vi "TCP-SV Message Interpreter.vi"(8 "error in (no error)":errorcluster, 9 "Data":variant, 10 "Message":string, 11 "Guardian in":refnum<class "Guardian.lvclass">) -> (0 "error out":errorcluster, 3 "Guardian out":refnum<class "Guardian.lvclass">)   [LabVIEW 2020, in "TALOS.lvlib" / "Guardian.lvlib" / "Guardian.lvclass"]
doc: "Use this VI to send a message to the Guardian, from the outside (i.e. from a uService). For internal messages, use the Actor Framework messages system."
uses:
  Guardian.lvclass
  C:/LabVIEW Code/TALOS/talos/Ancestor/Ancestor/Ancestor.lvclass
  C:/LabVIEW Code/TALOS/builds/Actor Framework PPL/Actor Framework.lvlibp/1abvi3w/vi.lib/ActorFramework/Actor/Actor.lvclass
  Ancestor/Ancestor/Ancestor.lvclass/Ancestor.ctl
  Father of all uServices/Father of all uServices/Event Handler Items.ctl
  Classes/uService List/uService List.lvclass/uService List.ctl
  Father of all uServices/Father of all uServices Messages/Event Handler Msg/Event Handler Msg.lvclass/Event Handler Msg.ctl
  Guardian Messages/Ready to launch Msg/Ready to launch Msg.lvclass/Ready to launch Msg.ctl
  Guardian.lvclass/Guardian.ctl
  Guardian Messages/Message to uService Msg/Message to uService Msg.lvclass/Message to uService Msg.ctl
  Ancestor/Ancestor/Infinite Message Selector.ctl
  Im alive message.ctl
  Guardian Messages/Message to Other Guardian Msg/Message to Other Guardian Msg.lvclass/Message to Other Guardian Msg.ctl
  Classes/uService List/Get Queue.vi
  FGV/Error Memory/Get Error Description.vi
  Support VIs/Get PC name.vi
  Support VIs/Get Class Name.vi
  <vilib>/Utility/error.llb/Clear Errors.vi
  Support VIs/Circus Root Path.vi
  FGV/Error Memory/Error Memory Core.vi
  <vilib>/AdvancedString/Delimited String to 1D String Array.vi
  FGV/Error Memory/Error Crt Lvl checker.vi
  FGV/Error Memory/Error Memory Core.vi/40c8088d-b597-4017-91af-faa98e00292e.vi
  FGV/Error Memory/Error Memory Core.vi/d4a3ab98-063c-4e44-b43d-fbdcfe6c2be2.vi
  Support VIs/Global Memory.vi
  <vilib>/Utility/LVClass/Get LV Class Name.vi
  Support VIs/TALOS Root path.vi
  Support VIs/Read CSV worksheet.vi
  Support VIs/Global Constants.vi
  <vilib>/Utility/error.llb/General Error Handler.vi
  <vilib>/Utility/config.llb/Open Config Data.vi
  <vilib>/Utility/config.llb/Get Section Names.vi
  <vilib>/Utility/config.llb/Get Key Names.vi
  <vilib>/Utility/config.llb/Read Key.vi
  <vilib>/Utility/config.llb/Read Key (String).vi
  <vilib>/Utility/config.llb/Close Config Data.vi
  builds/Actor Framework PPL/Actor Framework.lvlibp/1abvi3w/vi.lib/ActorFramework/Message Enqueuer/Enqueue.vi
  Support VIs/Error Log.vi
  Ancestor/Ancestor/Ancestor.lvclass
  <vilib>/Comparison/Equal/Equal Functor/Equal Functor.lvclass
  builds/Actor Framework PPL/Actor Framework.lvlibp/1abvi3w/vi.lib/ActorFramework/Message Enqueuer/Message Enqueuer.lvclass
  Father of all uServices/Father of all uServices Messages/Event Handler Msg/Event Handler Msg.lvclass
  Guardian Messages/Ready to launch Msg/Ready to launch Msg.lvclass
  Guardian Messages/Message to uService Msg/Message to uService Msg.lvclass
  Guardian Messages/Message to Other Guardian Msg/Message to Other Guardian Msg.lvclass
  Classes/Guardian List/Guardian List.lvclass
  Classes/Distributed uService Map/Distributed uService Map.lvclass
  TALOS.lvlib
  Father of all uServices/Father of all uServices/Father of all uServices.lvclass
  Classes/uService List/uService List.lvclass
  builds/Actor Framework PPL/Actor Framework.lvlibp/1abvi3w/vi.lib/ActorFramework/Actor/Actor.lvclass
  Classes/Error Filter/Error Filter.lvclass
  FGV/Error Memory/Error Memory.lvlib
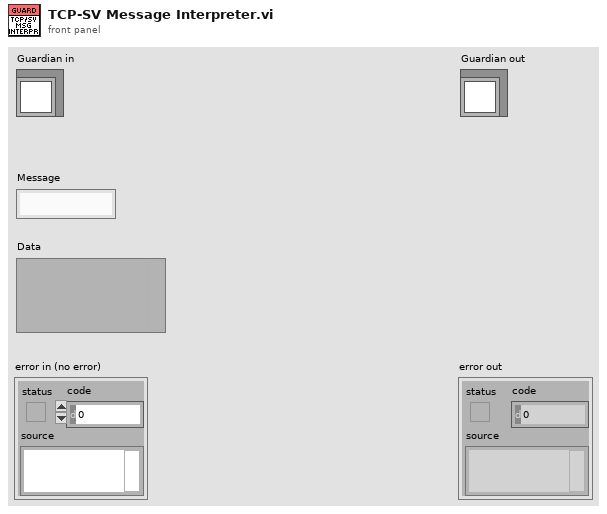
[diagram p1: front panel]
types:
  T1 = typedef "TALOS.lvlib/Father of all uServices.lvlib/Father of all uServices.lvclass/Event Handler Items.ctl" = enum16{"Button Pressed", "Shared Variable Updated", "Message", "Ready to launch?", "Safe Mode", "Start RUN", "Stop RUN"}
  T2 = typedef "TALOS.lvlib/Ancestor.lvlib/Ancestor.lvclass/Infinite Message Selector.ctl" = enum16{"Start", "Stop", "Check", "Flush (Stop all)", "Init"}
  T3 = typedef "TALOS.lvlib/Guardian.lvlib/Guardian.lvclass/Im alive message.ctl" = cluster{"ID":string, "Time":timestamp}
  T4 = cluster{"Accessors:ID":string, "All IDs":string[]}
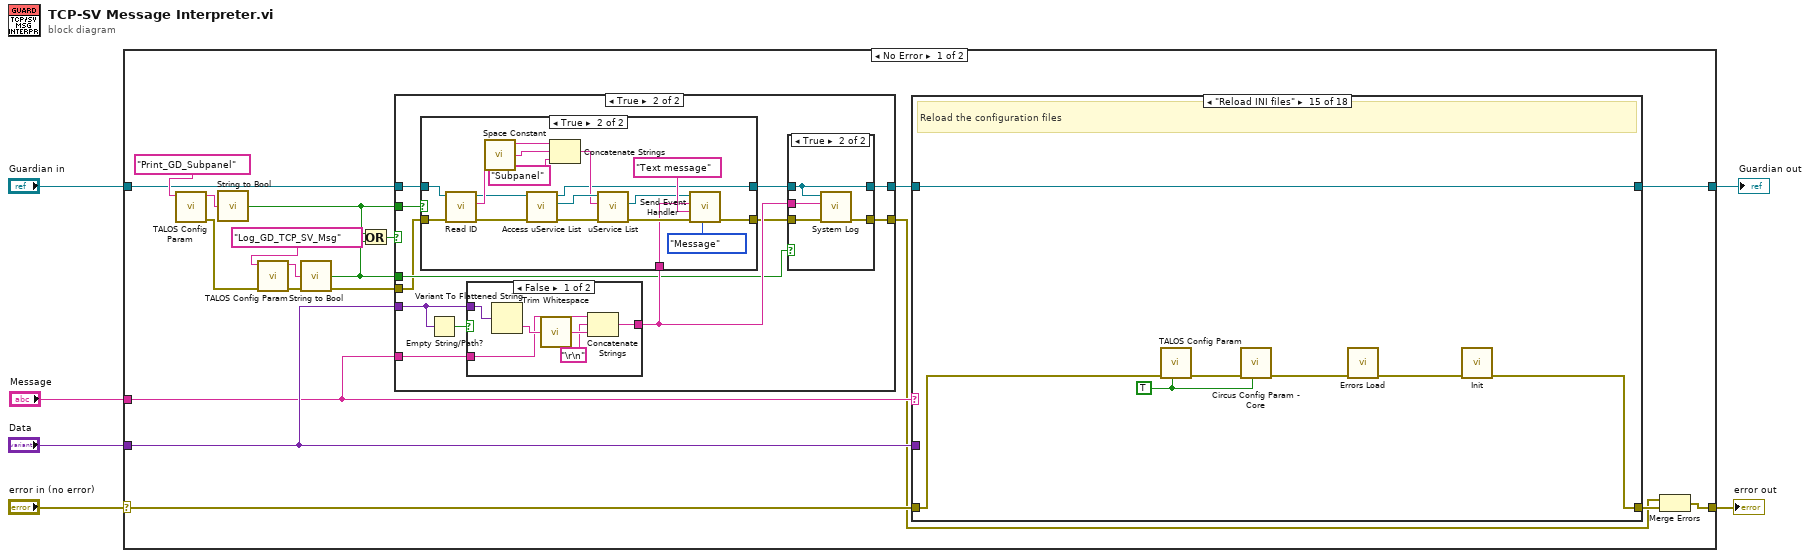
[diagram p0: block diagram]
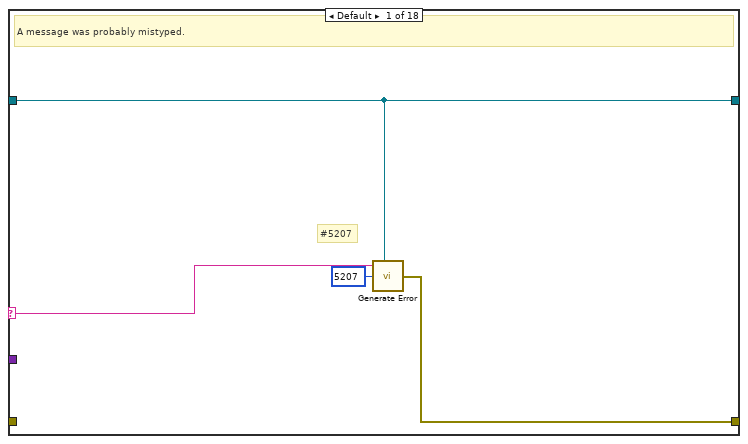
[diagram p6: hidden frame]
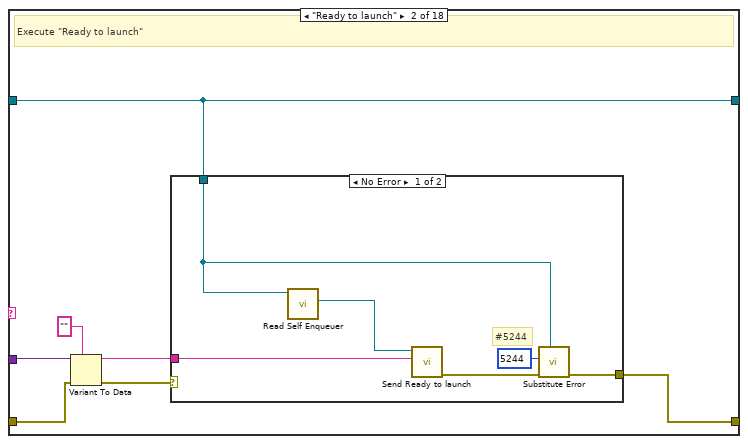
[diagram p7: hidden frame]
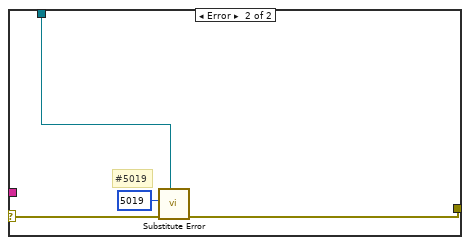
[diagram p8: hidden frame]
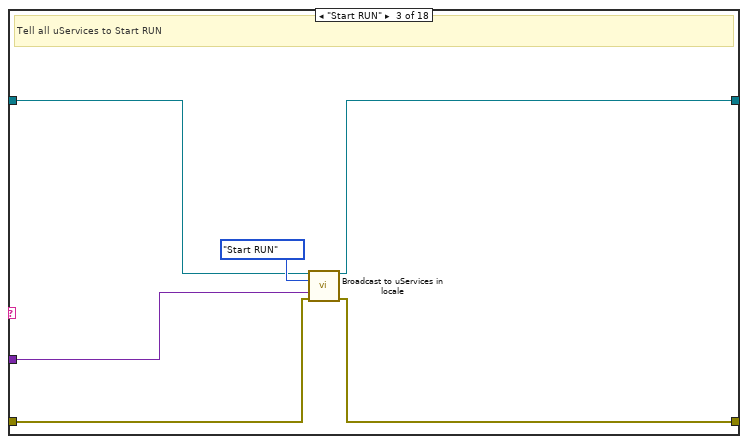
[diagram p9: hidden frame]
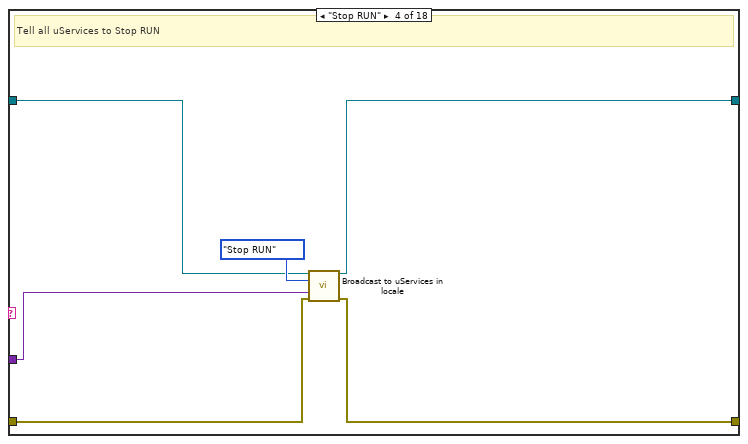
[diagram p10: hidden frame]
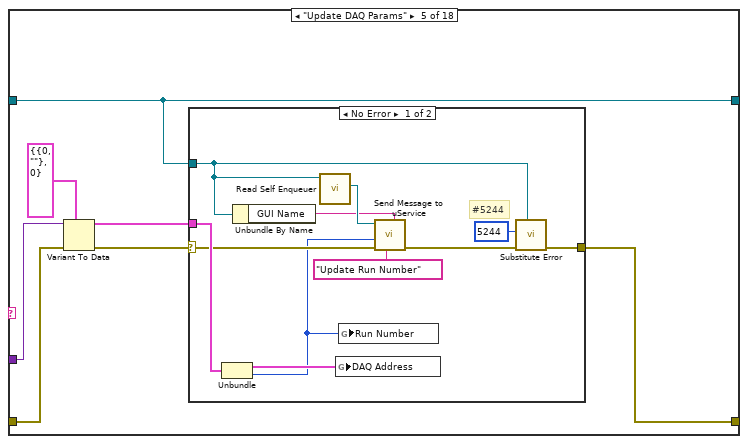
[diagram p11: hidden frame]
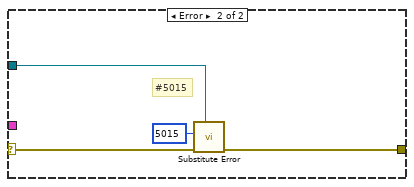
[diagram p12: hidden frame]
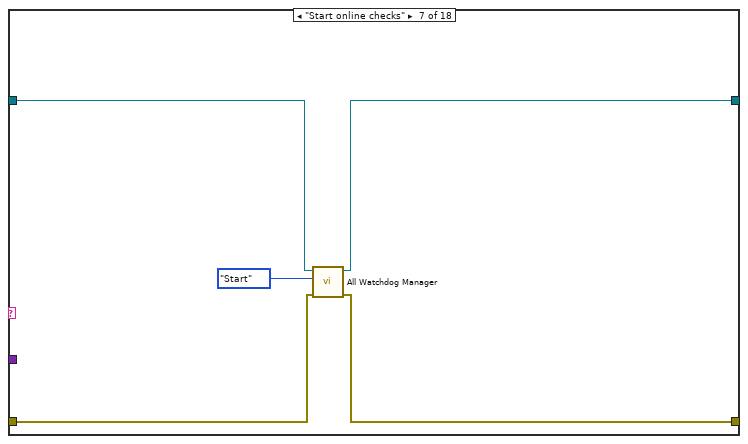
[diagram p14: hidden frame]
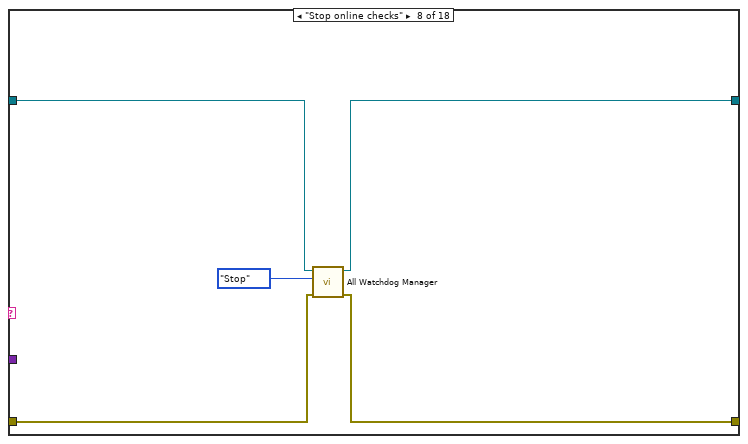
[diagram p15: hidden frame]
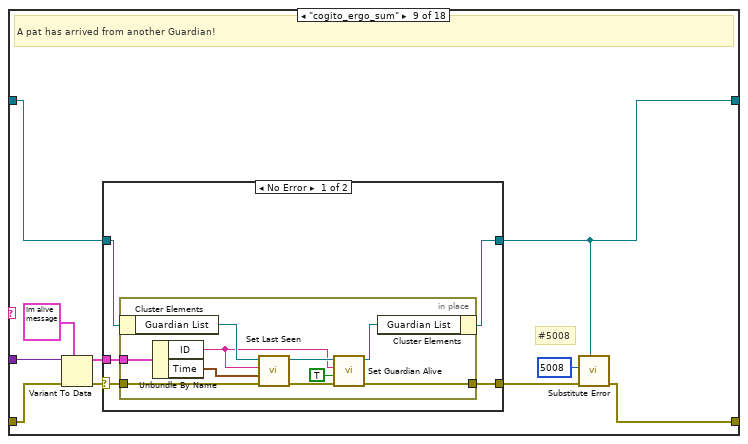
[diagram p16: hidden frame]
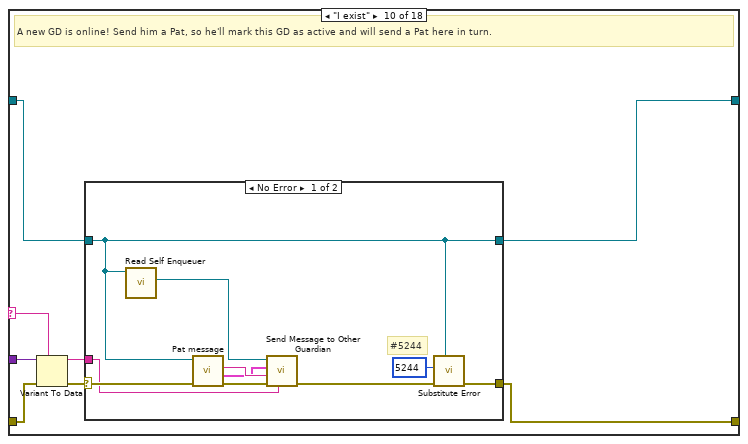
[diagram p18: hidden frame]
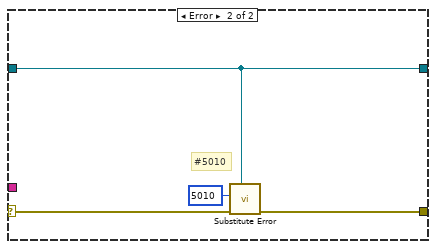
[diagram p19: hidden frame]
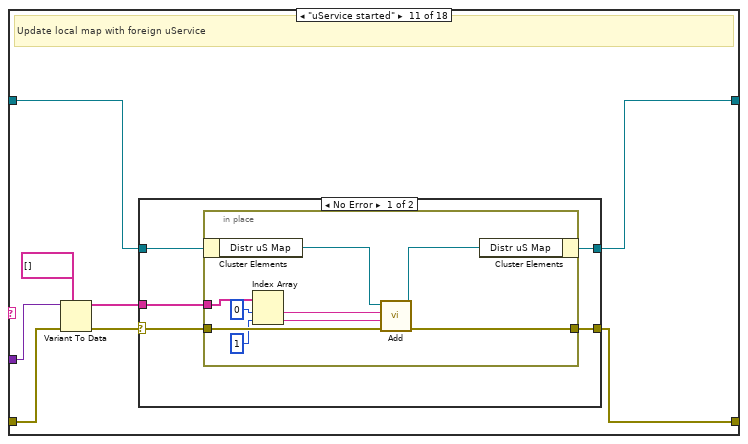
[diagram p20: hidden frame]
diagram:
  n1 = case shown="No Error" "error in (no error)" {
    selector: "error in (no error)" -> [w22 w358]
    tunnel: [w19 w358] -> w6
    tunnel: "Guardian in" -> [w15 w357]
    tunnel: [w23 w357] -> w3
    tunnel: "Data" -> [w21 _]
    tunnel: "Message" -> [w20 _]
    frame No Error {
      n2 = call "TALOS Config Param.vi"("Parameter Name"="Print_GD_Subpanel") -> ("error out"=w11:errorcluster, "Output"=w16:string)  [unwired: 9 in]
      n3 = call "String to Bool.vi"("String"=w16) -> ("Boolean"=w7:bool)
      n4 = call "TALOS Config Param.vi"("error in (no error)"=w11, "Parameter Name"="Log_GD_TCP_SV_Msg") -> ("error out"=w10:errorcluster, "Output"=w13:string)  [unwired: 8 in]
      n5 = call "String to Bool.vi"("String"=w13) -> ("Boolean"=w8:bool)
      n6 = Or(x=w7, y=w8) -> (x .or. y?=w9:bool)
      n7 = case shown="True" w9 {
        tunnel: w21 -> [_ w37]
        tunnel: w20 -> [_ w36]
        tunnel: [w25 w35] -> w18
        tunnel: w15 -> [w26 w31]
        tunnel: w7 -> [_ w30]
        tunnel: w8 -> [_ w29]
        tunnel: [w26 w28] -> w12
        tunnel: w10 -> [w25 w27]
        frame False {
        }
        frame True {
          n8 = Empty String/Path?(string/path=w37) -> (empty?=w38:bool)
          n9 = case shown="False" w38 {
            tunnel: w37 -> [w69 _]
            tunnel: w36 -> [w66 w70]
            tunnel: [w64 w70] -> w34
            frame False {
              n10 = Variant To Flattened String(Variant=w69) -> (data string=w68:string)  [unwired: 1 out]
              n11 = call <vilib>:"Trim Whitespace.vi"("string"=w68) -> ("trimmed string"=w67:string)  [unwired: 1 in]
              n12 = Concatenate Strings(w66, "\r\n", w67) -> (w64:string)
            }
            frame True {
            }
          }
          n13 = case shown="True" w30 {
            tunnel: w34 -> [_ w54]
            tunnel: [w40 w47] -> w33
            tunnel: [w39 w46] -> w32
            tunnel: w31 -> [w40 w43]
            tunnel: w27 -> [w39 w42]
            frame False {
            }
            frame True {
              n14 = call "Read ID.vi"("error in (no error)"=w42, "Ancestor in"=w43) -> ("error out"=w41:errorcluster, "ID"=w45:string, "Ancestor out"=w44:refnum<class "Guardian.lvclass">)  [unwired: 7 in]
              n15 = call <vilib>:"Space Constant.vi"() -> ("String"=w48:string)
              n16 = call-dynamic "Access uService List.vi"("error in (no error)"=w41, "Ancestor in"=w44) -> ("error out"=w52:errorcluster, "uService List out"=w51:refnum<class "uService List.lvclass">, "Ancestor out"=w47:refnum<class "Guardian.lvclass">)  [unwired: 7 in]
              n17 = Concatenate Strings(w45, w48, "Subpanel" ("string")) -> (w50:string)
              n18 = call-poly "uService List.vi"("error in (no error)"=w52, "ID"=w50, "uService List in"=w51) -> ("error out"=w57:errorcluster, "uService Queue"=w53:refnum<class "Message Enqueuer.lvclass">)  [unwired: 6 in, 1 out]
              n19 = call "Send Event Handler.vi"("Event type"=Event_Handler_Items."Message", "error in (no error)"=w57, "Item Name"="Text message" ("Message"), "Data"=w54, "Message Enqueuer"=w53) -> ("error out"=w46:errorcluster)  [unwired: 5 in, 1 out]
            }
          }
          n20 = case shown="True" w29 {
            tunnel: [w59 w63] -> w35
            tunnel: w34 -> [_ w62]
            tunnel: w33 -> [w58 w60]
            tunnel: w32 -> [w59 w61]
            tunnel: [w58 w60] -> w28
            frame False {
            }
            frame True {
              n21 = call "System Log.vi"("error in (no error)"=w61, "Text to log"=w62, "Object in"=w60) -> ("error out"=w63:errorcluster)  [unwired: 8 in]
            }
          }
        }
      }
      n22 = case shown="\"Reload INI files\"" w20 {
        selector: w20 -> [w72 _ _ _ _ _ _ _ _ w166 _ _ _ _ _ w316 _ _]
        tunnel: [w73 w80 w95 w101 w105 w126 w129 w134 w139 w165 w187 w213 w239 w268 w302 w310 w324 w349] -> w24
        tunnel: w21 -> [_ w79 w92 w98 w110 _ _ _ w147 w172 w192 w218 w244 w272 _ w314 _ w356]
        tunnel: w12 -> [w71 w81 w93 w99 w106 w127 w132 w137 w142 w168 w194 w220 w246 w274 w308 w309 w323 w347]
        tunnel: [w71 w81 w96 w102 w106 w127 w131 w136 w140 w167 w193 w219 w245 w273 w308 w309 w321 w348] -> w23
        tunnel: w22 -> [_ w78 w94 w100 w104 w126 w128 w133 w145 w171 w191 w217 w243 w271 w307 w313 w325 w350]
        frame Default {
          # "#5207"
          # "A message was probably mistyped."
          n23 = call "Generate Error.vi"("Optional String"=w72, "Class"=w71, "Error Code"=5207) -> ("error out"=w73:errorcluster)  [unwired: 4 in]
        }
        frame "Ready to launch" {
          # "Execute \"Ready to launch\""
          n24 = Variant To Data(error in=w78, type="", Variant=w79) -> (data=w75:string, error out=w76:errorcluster)
          n25 = case shown="No Error" w76 {
            selector: w76 -> [_ w90]
            tunnel: w81 -> [w82 w91]
            tunnel: [w83 w89] -> w80
            tunnel: w75 -> [w86 _]
            frame No Error {
              # "#5244"
              n26 = call "Read Self Enqueuer.vi"("Actor"=w82) -> ("Self Enqueuer"=w87:refnum<class "Message Enqueuer.lvclass">)  [unwired: 10 in]
              n27 = call "Send Ready to launch.vi"("GUID"=w86, "Message Enqueuer"=w87) -> ("error out"=w84:errorcluster)  [unwired: 8 in, 1 out]
              n28 = call "Substitute Error.vi"("LabVIEW Object"=w82, "error in (no error)"=w84, "Error Code"=5244) -> ("error out"=w83:errorcluster)  [unwired: 8 in]
            }
            frame Error {
              # "#5019"
              n29 = call "Substitute Error.vi"("LabVIEW Object"=w91, "error in (no error)"=w90, "Error Code"=5019) -> ("error out"=w89:errorcluster)  [unwired: 8 in]
            }
          }
        }
        frame "Start RUN" {
          # "Tell all uServices to Start RUN"
          n30 = call "Broadcast to uServices in locale.vi"("Guardian in"=w93, "Event type"=Event_Handler_Items."Start RUN", "Data"=w92, "error in (no error)"=w94) -> ("Guardian out"=w96:refnum<class "Guardian.lvclass">, "error out"=w95:errorcluster)  [unwired: 10 in]
        }
        frame "Stop RUN" {
          # "Tell all uServices to Stop RUN"
          n31 = call "Broadcast to uServices in locale.vi"("Guardian in"=w99, "Event type"=Event_Handler_Items."Stop RUN", "Data"=w98, "error in (no error)"=w100) -> ("Guardian out"=w102:refnum<class "Guardian.lvclass">, "error out"=w101:errorcluster)  [unwired: 10 in]
        }
        frame "Update DAQ Params" {
          n32 = Variant To Data(error in=w104, type=cluster{cluster{u16, string}, i32} {{0, ""}, 0}, Variant=w110) -> (data=w108:cluster{cluster{u16, string}, i32}, error out=w107:errorcluster)
          n33 = case shown="No Error" w107 {
            selector: w107 -> [w118 w125]
            tunnel: w108 -> [w119 _]
            tunnel: w106 -> [w112 w123]
            tunnel: [w111 w124] -> w105
            frame No Error {
              # "#5244"
              n34 = Unbundle(w119) -> (w116:cluster{u16, string}, w115:i32)
              n35 = Unbundle By Name(w112) -> ("GUI Name"=w120:string)
              n36 = call "Read Self Enqueuer.vi"("Actor"=w112) -> ("Self Enqueuer"=w121:refnum<class "Message Enqueuer.lvclass">)  [unwired: 10 in]
              n37 = global write "Global Memory.vi" "DAQ Address"(w116) -> ()
              n38 = global write "Global Memory.vi" "Run Number"(w115) -> ()
              n39 = call "Send Message to uService.vi"("uService ID"=w120, "Message"="Update Run Number", "error in (no error)"=w118, "Data"=w115, "Message Enqueuer"=w121) -> ("error out"=w113:errorcluster)  [unwired: 5 in, 1 out]
              n40 = call "Substitute Error.vi"("LabVIEW Object"=w112, "error in (no error)"=w113, "Error Code"=5244) -> ("error out"=w111:errorcluster)  [unwired: 8 in]
            }
            frame Error {
              # "#5015"
              n41 = call "Substitute Error.vi"("LabVIEW Object"=w123, "error in (no error)"=w125, "Error Code"=5015) -> ("error out"=w124:errorcluster)  [unwired: 8 in]
            }
          }
        }
        frame "Text Message" {
          # "For testing purpouses"
        }
        frame "Start online checks" {
          n42 = call "All Watchdog Manager.vi"("error in (no error)"=w128, "Infinite Message Selector"=Infinite_Message_Selector."Start", "Guardian in"=w132) -> ("error out"=w129:errorcluster, "Guardian out"=w131:refnum<class "Guardian.lvclass">)  [unwired: 6 in, 1 out]
        }
        frame "Stop online checks" {
          n43 = call "All Watchdog Manager.vi"("error in (no error)"=w133, "Infinite Message Selector"=Infinite_Message_Selector."Stop", "Guardian in"=w137) -> ("error out"=w134:errorcluster, "Guardian out"=w136:refnum<class "Guardian.lvclass">)  [unwired: 6 in, 1 out]
        }
        frame "cogito_ergo_sum" {
          # "#5008"
          # "A pat has arrived from another Guardian!"
          n44 = Variant To Data(error in=w145, type=T3 {"ID"="", "Time"=timestamp(0 s since 1904-01-01)} ("cluster"), Variant=w147) -> (data=w144:T3, error out=w143:errorcluster)
          n45 = case shown="No Error" w143 {
            selector: w143 -> [w149 w163]
            tunnel: w144 -> [w150 _]
            tunnel: w142 -> [w152 w164]
            tunnel: [w151 w164] -> w140
            tunnel: [w148 w163] -> w141
            frame No Error {
              n46 = in-place {
                in-place-border: w150 -> [w161]
                in-place-border: w149 -> [w159]
                in-place-border: [w155] -> w148
                n47 = in-place-cluster #1(w152) -> ("Guardian List"=w162:refnum<class "Guardian List.lvclass">)
                n48 = Unbundle By Name(w161) -> ("ID"=w154:string, "Time"=w160:timestamp)
                n49 = call-dynamic "Set Last Seen.vi"("error in (no error)"=w159, "Last Seen"=w160, "ID"=w154, "Guardian List in"=w162) -> ("error out"=w156:errorcluster, "Guardian List out"=w158:refnum<class "Guardian List.lvclass">)  [unwired: 6 in]
                n50 = call-dynamic "Set Guardian Alive.vi"("error in (no error)"=w156, "Alive"=TRUE, "ID"=w154, "Guardian List in"=w158) -> ("error out"=w155:errorcluster, "Guardian List out"=w157:refnum<class "Guardian List.lvclass">)  [unwired: 6 in]
                n51 = in-place-cluster #1("Guardian List"=w157) -> (w151:refnum<class "Guardian.lvclass">)
              }
            }
            frame Error {
            }
          }
          n52 = call "Substitute Error.vi"("LabVIEW Object"=w140, "error in (no error)"=w141, "Error Code"=5008) -> ("error out"=w139:errorcluster)  [unwired: 8 in]
        }
        frame "I exist" {
          # "A new GD is online! Send him a Pat, so he'll mark this GD as active and will send a Pat here in turn."
          n53 = Variant To Data(error in=w171, type=w166, Variant=w172) -> (data=w170:string, error out=w169:errorcluster)
          n54 = case shown="No Error" w169 {
            selector: w169 -> [w181 w185]
            tunnel: w170 -> [w180 _]
            tunnel: w168 -> [w174 w186]
            tunnel: [w174 w186] -> w167
            tunnel: [w173 w183] -> w165
            frame No Error {
              # "#5244"
              n55 = call "Read Self Enqueuer.vi"("Actor"=w174) -> ("Self Enqueuer"=w182:refnum<class "Message Enqueuer.lvclass">)  [unwired: 10 in]
              n56 = call "Pat message.vi"("error in (no error)"=w181, "Guardian in"=w174) -> ("error out"=w177:errorcluster, "Data"=w178:T3, "Message name"=w179:string)  [unwired: 6 in, 1 out]
              n57 = call "Send Message to Other Guardian.vi"("Guardian ID"=w180, "error in (no error)"=w177, "Message"=w179, "Data"=w178, "Message Enqueuer"=w182) -> ("error out"=w175:errorcluster)  [unwired: 5 in, 1 out]
              n58 = call "Substitute Error.vi"("LabVIEW Object"=w174, "error in (no error)"=w175, "Error Code"=5244) -> ("error out"=w173:errorcluster)  [unwired: 8 in]
            }
            frame Error {
              # "#5010"
              n59 = call "Substitute Error.vi"("LabVIEW Object"=w186, "error in (no error)"=w185, "Error Code"=5010) -> ("error out"=w183:errorcluster)  [unwired: 8 in]
            }
          }
        }
        frame "uService started" {
          # "Update local map with foreign uService"
          n60 = Variant To Data(error in=w191, type=string[] [], Variant=w192) -> (data=w188:string[], error out=w189:errorcluster)
          n61 = case shown="No Error" w189 {
            selector: w189 -> [w197 w212]
            tunnel: w194 -> [w199 w210]
            tunnel: [w198 w210] -> w193
            tunnel: w188 -> [w195 _]
            tunnel: [w196 w209] -> w187
            frame No Error {
              n62 = in-place {
                in-place-border: w197 -> [w206]
                in-place-border: [w205] -> w196
                in-place-border: w195 -> [w204]
                n63 = in-place-cluster #2(w199) -> ("Distr uS Map"=w208:refnum<class "Distributed uService Map.lvclass">)
                n64 = Index Array(array=w204, index #1=0 ("index"), index #2=1 ("index")) -> (element #1=w201:string, element #2=w200:string)
                n65 = call-dynamic "Add.vi"("error in (no error)"=w206, "uService"=w200, "Guardian"=w201, "Distributed uService Map in"=w208) -> ("error out"=w205:errorcluster, "Distributed uService Map out"=w207:refnum<class "Distributed uService Map.lvclass">)  [unwired: 5 in, 1 out]
                n66 = in-place-cluster #2("Distr uS Map"=w207) -> (w198:refnum<class "Guardian.lvclass">)
              }
            }
            frame Error {
              # "#5102"
              n67 = call "Substitute Error.vi"("LabVIEW Object"=w210, "error in (no error)"=w212, "Error Code"=5102) -> ("error out"=w209:errorcluster)  [unwired: 8 in]
            }
          }
        }
        frame "uService stopped" {
          # "Update local map with foreign uService"
          n68 = Variant To Data(error in=w217, type=string[] [], Variant=w218) -> (data=w214:string[], error out=w215:errorcluster)
          n69 = case shown="No Error" w215 {
            selector: w215 -> [w223 w238]
            tunnel: w220 -> [w225 w236]
            tunnel: [w224 w236] -> w219
            tunnel: w214 -> [w221 _]
            tunnel: [w222 w235] -> w213
            frame No Error {
              n70 = in-place {
                in-place-border: w223 -> [w232]
                in-place-border: [w231] -> w222
                in-place-border: w221 -> [w230]
                n71 = in-place-cluster #3(w225) -> ("Distr uS Map"=w234:refnum<class "Distributed uService Map.lvclass">)
                n72 = Index Array(array=w230, index #1=0 ("index"), index #2=1 ("index")) -> (element #1=w227:string, element #2=w226:string)
                n73 = call-dynamic "Remove.vi"("error in (no error)"=w232, "uService ID"=w226, "Guardian"=w227, "Distributed uService Map in"=w234) -> ("error out"=w231:errorcluster, "Distributed uService Map out"=w233:refnum<class "Distributed uService Map.lvclass">)  [unwired: 5 in, 1 out]
                n74 = in-place-cluster #3("Distr uS Map"=w233) -> (w224:refnum<class "Guardian.lvclass">)
              }
            }
            frame Error {
              # "#5102"
              n75 = call "Substitute Error.vi"("LabVIEW Object"=w236, "error in (no error)"=w238, "Error Code"=5102) -> ("error out"=w235:errorcluster)  [unwired: 8 in]
            }
          }
        }
        frame "Get uService List" {
          # "Give to the requesting Guardian the current uService List (for initialise the distributed one)"
          n76 = Variant To Data(error in=w243, type="", Variant=w244) -> (data=w240:string, error out=w241:errorcluster)
          n77 = case shown="No Error" w241 {
            selector: w241 -> [w257 w266]
            tunnel: w246 -> [w258 w264]
            tunnel: [w247 w264] -> w245
            tunnel: w240 -> [w262 _]
            tunnel: [w248 w263] -> w239
            frame No Error {
              # "#5244"
              # "requesting GD"
              n78 = call-dynamic "Access uService List.vi"("error in (no error)"=w257, "Ancestor in"=w258) -> ("error out"=w255:errorcluster, "uService List out"=w256:refnum<class "uService List.lvclass">, "Ancestor out"=w259:refnum<class "Guardian.lvclass">)  [unwired: 7 in]
              n79 = call "Get all IDs.vi"("error in (no error)"=w255, "uService List"=w256) -> ("error out"=w254:errorcluster, "All IDs"=w252:string[])  [unwired: 7 in, 1 out]
              n80 = property class="Guardian.lvclass"(reference=w259) -> (reference out=w247:refnum<class "Guardian.lvclass">, "Accessors:ID"=w253:string)  [unwired: 1 in, 1 out]
              n81 = Bundle("Accessors:ID"=w253, "All IDs"=w252) -> (w251:T4)  [unwired: 1 in]
              n82 = call "Read Self Enqueuer.vi"("Actor"=w247) -> ("Self Enqueuer"=w261:refnum<class "Message Enqueuer.lvclass">)  [unwired: 10 in]
              n83 = call "Send Message to Other Guardian.vi"("Guardian ID"=w262, "error in (no error)"=w254, "Message"="Current uService List", "Data"=w251, "Message Enqueuer"=w261) -> ("error out"=w249:errorcluster)  [unwired: 5 in, 1 out]
              n84 = call "Substitute Error.vi"("LabVIEW Object"=w247, "error in (no error)"=w249, "Error Code"=5244) -> ("error out"=w248:errorcluster)  [unwired: 8 in]
            }
            frame Error {
              # "#5102"
              n85 = call "Substitute Error.vi"("LabVIEW Object"=w264, "error in (no error)"=w266, "Error Code"=5102) -> ("error out"=w263:errorcluster)  [unwired: 8 in]
            }
          }
        }
        frame "Current uService List" {
          # "Update Distributed uService List with the list received"
          n86 = Variant To Data(error in=w271, type=cluster{"String":string, string[]} {"String"="", []}, Variant=w272) -> (data=w269:cluster{"String":string, string[]}, error out=w270:errorcluster)
          n87 = case shown="No Error" w270 {
            selector: w270 -> [w277 w301]
            tunnel: w274 -> [w279 w299]
            tunnel: [w275 w299] -> w273
            tunnel: w269 -> [w278 _]
            tunnel: [w276 w298] -> w268
            frame No Error {
              n88 = in-place {
                in-place-border: w278 -> [w289]
                in-place-border: w277 -> [w287]
                in-place-border: [w282] -> w276
                n89 = in-place-cluster #4(w279) -> ("Distr uS Map"=w291:refnum<class "Distributed uService Map.lvclass">, "Guardian List"=w284:refnum<class "Guardian List.lvclass">)
                n90 = Unbundle(w289) -> ("String"=w285:string, w288:string[])
                n91 = for {
                  shift-right: [w296] -> w290
                  shift-left: w291 -> [w297]
                  tunnel: w285 -> [w295]
                  tunnel: w288 -> [w294] mode=indexing
                  shift-right: [w292] -> w286
                  shift-left: w287 -> [w293]
                  n92 = call-dynamic "Add.vi"("error in (no error)"=w293, "uService"=w294, "Guardian"=w295, "Distributed uService Map in"=w297) -> ("error out"=w292:errorcluster, "Distributed uService Map out"=w296:refnum<class "Distributed uService Map.lvclass">)  [unwired: 5 in, 1 out]
                }
                n93 = call-dynamic "Set uS List Received.vi"("uS List Received"=TRUE, "ID"=w285, "Guardian List in"=w284) -> ("error out"=w281:errorcluster, "Guardian List out"=w283:refnum<class "Guardian List.lvclass">)  [unwired: 7 in]
                n94 = in-place-cluster #4("Distr uS Map"=w290, "Guardian List"=w283) -> (w275:refnum<class "Guardian.lvclass">)
                n95 = Merge Errors(w286, w281) -> (w282:errorcluster)
              }
            }
            frame Error {
              # "#5102"
              n96 = call "Substitute Error.vi"("LabVIEW Object"=w299, "error in (no error)"=w301, "Error Code"=5102) -> ("error out"=w298:errorcluster)  [unwired: 8 in]
            }
          }
        }
        frame "Reload INI files" {
          w305 = TRUE ("Load")
          # "Reload the configuration files"
          n97 = call "TALOS Config Param.vi"("Load"=w305, "error in (no error)"=w307) -> ("error out"=w306:errorcluster)  [unwired: 8 in, 1 out]
          n98 = call "Circus Config Param - Core.vi"("Load"=w305, "error in (no error)"=w306) -> ("error out"=w304:errorcluster)  [unwired: 8 in, 1 out]
          n99 = call "Errors Load.vi"("error in (no error)"=w304) -> ("error out"=w303:errorcluster)  [unwired: 10 in]
          n100 = call "Init.vi"("error in (no error)"=w303) -> ("error out"=w302:errorcluster)  [unwired: 10 in]
        }
        frame "Change Run LED color", "Reset Run LED", "Run Stopped with Errors", "Update Error Listbox", "Update Kasli Log", "Update Run Status" {
          # "#5244"
          n101 = Unbundle By Name(w309) -> ("GUI Name"=w317:string)
          n102 = call "Read Self Enqueuer.vi"("Actor"=w309) -> ("Self Enqueuer"=w318:refnum<class "Message Enqueuer.lvclass">)  [unwired: 10 in]
          n103 = call "Send Message to uService.vi"("uService ID"=w317, "Message"=w316, "error in (no error)"=w313, "Data"=w314, "Locale?"=TRUE, "Message Enqueuer"=w318) -> ("error out"=w311:errorcluster)  [unwired: 4 in, 1 out]
          n104 = call "Substitute Error.vi"("LabVIEW Object"=w309, "error in (no error)"=w311, "Error Code"=5244) -> ("error out"=w310:errorcluster)  [unwired: 8 in]
        }
        frame "Update from GIT" {
          n105 = flat-sequence {
            tunnel: w325 -> [_]
            tunnel: [w326] -> w319
            tunnel: w323 -> [w331]
            tunnel: [w330] -> w320
            tunnel: w323 -> [w345]
            tunnel: [w344] -> w322
            tunnel: [w343] -> w321
            frame #0 {
              n106 = for {
                tunnel: i32[] [5004, 5005] ("Error Code") -> [w329] mode=indexing
                tunnel: [w328] -> w326 mode=indexing
                n107 = call "Add.vi"("Error Code"=w329) -> ("error out"=w328:errorcluster)  [unwired: 10 in]
              }
            }
            frame #1 {
              n108 = global read "Global Constants.vi" "Local"() -> (w335:bool)
              n109 = call "Is in Packed Library.vi"() -> ("error out"=w336:errorcluster, "Is In Packed Library"=w333:bool)  [unwired: 10 in]
              n110 = Not(x=w333) -> (.not. x?=w334:bool)
              n111 = Or(x=w335, y=w334) -> (x .or. y?=w332:bool)
              n112 = case shown="False" w332 {
                tunnel: w336 -> [w339 w342]
                tunnel: [w338 w341] -> w330
                tunnel: w331 -> [w337 _]
                frame False {
                  n113 = call "Launch Update from Git.vi"("error in (no error)"=w339, "Guardian in"=w337) -> ("error out"=w338:errorcluster)  [unwired: 8 in, 1 out]
                }
                frame True {
                  n114 = call "Temporised Pop-up Window.vi"("error in (no error)"=w342, "Text"="I'm dying!") -> ("error out"=w341:errorcluster)  [unwired: 9 in]
                }
              }
            }
            frame #2 {
              n115 = call "System shutdown.vi"("Guardian in"=w345) -> ("error out"=w344:errorcluster, "Guardian out"=w343:refnum<class "Guardian.lvclass">)  [unwired: 9 in]
            }
          }
          n116 = Merge Errors(w322, w320, w319) -> (w324:errorcluster)
        }
        frame "uServices Safe Mode" {
          w354 = TRUE
          n117 = Variant To Data(type=w354, Variant=w356) -> (data=w353:bool, error out=w355:errorcluster)  [unwired: 1 in]
          n118 = Select(t=w354, s=w355, f=w353) -> (s? t:f=w351:bool)
          n119 = call "Broadcast to uServices in locale.vi"("Guardian in"=w347, "Event type"=Event_Handler_Items."Safe Mode", "Message"="Safe Mode!", "Data"=w351, "error in (no error)"=w350) -> ("Guardian out"=w348:refnum<class "Guardian.lvclass">, "error out"=w349:errorcluster)  [unwired: 9 in]
        }
      }
      n120 = Merge Errors(w18, w24) -> (w19:errorcluster)
    }
    frame Error {
    }
  }
  "error out" <- w6
  "Guardian out" <- w3
